vi "4000 Compatible.vi"() -> ()   [LabVIEW 2017]
panel:
  out "4000 compatible?":bool=TRUE
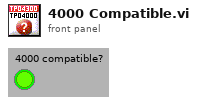
[diagram p1: front panel]
diagram:
